vi "Get Waveform.vi"(8 "error in (no error)":errorcluster, 10 "Save data":bool, 11 "Tektronix Driver in":refnum<class "Tektronix 4000 Driver.lvclass">) -> (0 "error out":errorcluster, 2 "Waveform":waveform(dbl), 3 "Tektronix Driver out":refnum<class "Tektronix 4000 Driver.lvclass">)   [LabVIEW 2021, in "Tektronix 4000 Driver.lvclass"]
uses:
  Tektronix 4000 Driver.lvclass
  C:/GitHub/NHMFL_Core/Libraries/Instruments/Tektronix/Tektronix Driver/Tektronix Driver.lvclass
  Tektronix 4000 Driver.lvclass/Tektronix 4000 Driver.ctl
  <instrlib>/Tektronix DPO MSO 2000 4000 Series/Public/Data/Read (Single Waveform).vi
  <instrlib>/Tektronix DPO MSO 2000 4000 Series/Tektronix DPO MSO 2000 4000 Series.lvlib
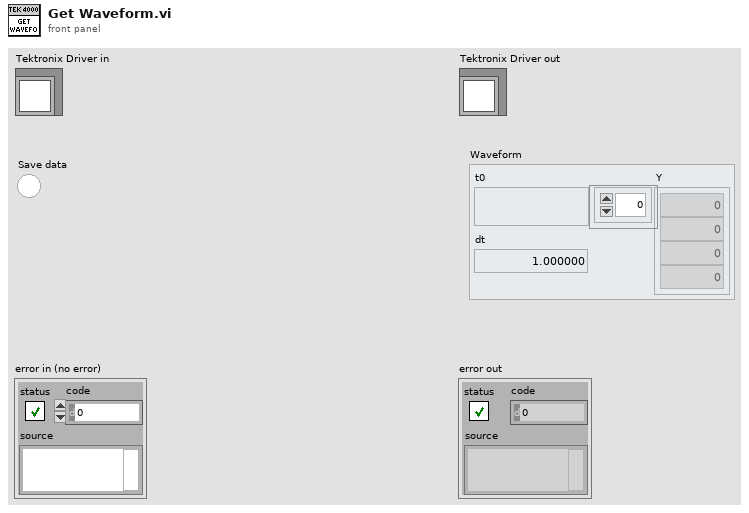
[diagram p1: front panel]
types:
  T1 = typedef "Tektronix Configuration.ctl" = cluster{"Channel":i32, "Number of averages":i32, "Input impedace":enum16{"1 M Ohm", "50 Ohm"}, "Vertical coupling":enum16{"AC", "DC", "Ground"}}
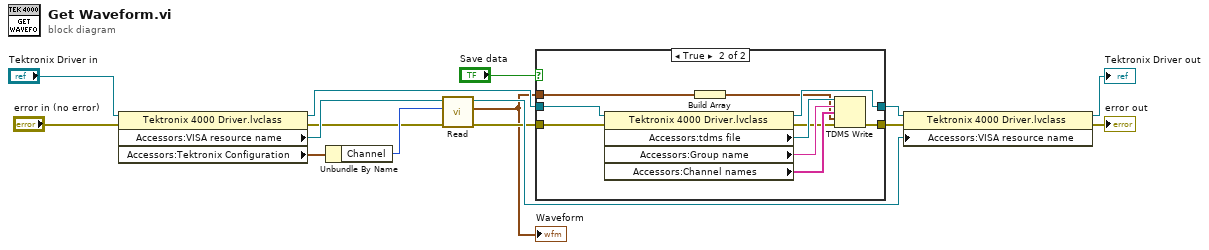
[diagram p0: block diagram]
diagram:
  n1 = property class="Tektronix 4000 Driver.lvclass"(reference="Tektronix Driver in", error in="error in (no error)") -> (reference out=w6:refnum<class "Tektronix 4000 Driver.lvclass">, error out=w9:errorcluster, "Accessors:VISA resource name"=w10:refnum<visa-resource-name>, "Accessors:Tektronix Configuration"=w15:T1)
  n2 = Unbundle By Name(w15) -> ("Channel"=w11:i32)
  n3 = call-poly <instrlib>:"Read.vi"("error in (no error)"=w9, "Channel (0: Channel 1)"=w11, "VISA resource name"=w10) -> ("error out"=w4:errorcluster, "Waveform Graph"=w3:waveform(dbl), "VISA resource name out"=w8:refnum<visa-resource-name>)  [unwired: 6 in]
  "Waveform" <- w3
  n4 = case shown="True" "Save data" {
    tunnel: w6 -> [w17 w26]
    tunnel: [w17 w27] -> w5
    tunnel: w4 -> [w16 w25]
    tunnel: w3 -> [_ w21]
    tunnel: [w16 w18] -> w2
    frame False {
    }
    frame True {
      n5 = property class="Tektronix 4000 Driver.lvclass"(reference=w26, error in=w25) -> (reference out=w27:refnum<class "Tektronix 4000 Driver.lvclass">, error out=w19:errorcluster, "Accessors:tdms file"=w24:refnum<k34>, "Accessors:Group name"=w23:string, "Accessors:Channel names"=w22:string[])
      n6 = Build Array(w21) -> (w20:waveform(dbl)[])
      n7 = TDMS Write(0:w24, 5:w23, 7:w22, 9:w20, 11:w19) -> (15:w18:errorcluster)  [unwired: 1 in, 3 out]
    }
  }
  n8 = property class="Tektronix 4000 Driver.lvclass"(reference=w5, error in=w2, "Accessors:VISA resource name"=w8) -> (reference out=→"Tektronix Driver out":refnum<class "Tektronix 4000 Driver.lvclass">, error out=→"error out":errorcluster)
